vi "Retrieve trace.vi"(5 "max points":i32, 7 "Data.PG in":refnum<class "Data.PG.lvclass">, 8 "error in (no error)":errorcluster, 9 "path table:column":string, 10 "End":timestamp, 11 "Start":timestamp) -> (0 "error out":errorcluster, 2 "Trace":cluster{timestamp[], dbl[]}, 3 "Data.PG out":refnum<class "Data.PG.lvclass">)   [LabVIEW 2020, in "Data.PG.lvclass"]
uses:
  Data.PG.lvclass
  <vilib>/Utility/error.llb/Error Cluster From Error Code.vi
  <vilib>/ErrorRing/Error Ring.xnode
panel:
  out "resulting string":string
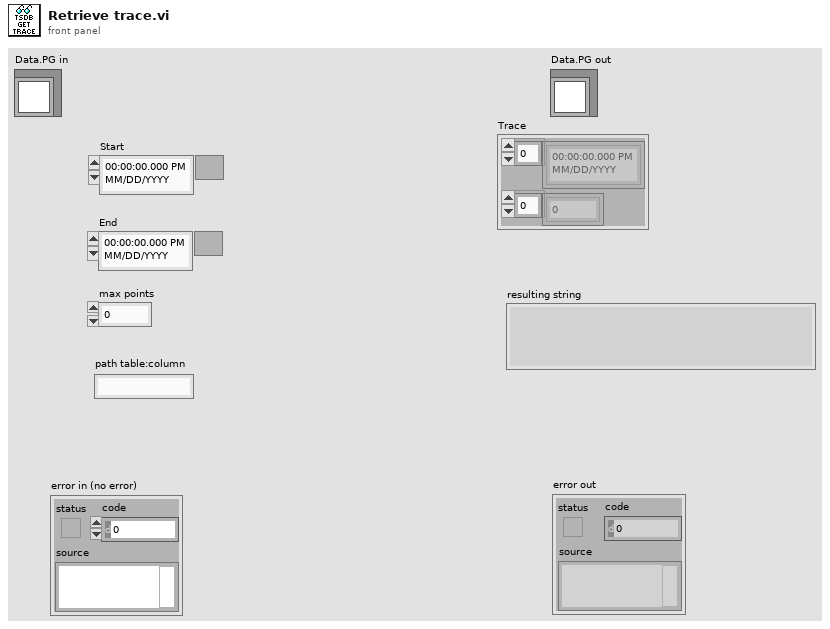
[diagram p1: front panel]
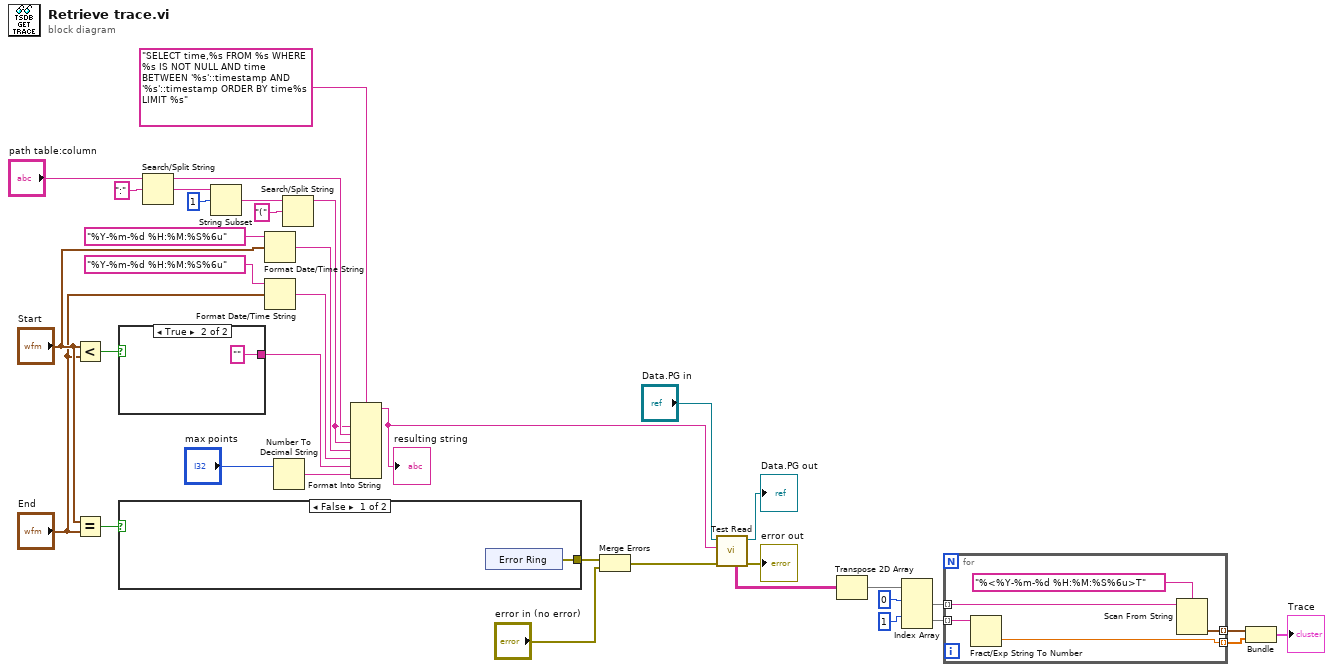
[diagram p0: block diagram]
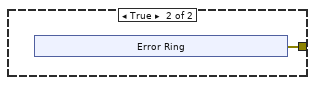
[diagram p2: hidden frame]
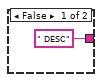
[diagram p3: hidden frame]
diagram:
  n1 = Less?(x="Start", y="End") -> (x < y?=w33:bool)
  n2 = Equal?(x="Start", y="End") -> (x = y?=w32:bool)
  n3 = case shown="True" w33 {
    tunnel: [" DESC" ""] -> w11
    frame False {
    }
    frame True {
    }
  }
  n4 = case shown="False" w32 {
    tunnel: [w39 w41] -> w31
    frame False {
      n5 = xnode "Error Ring"() -> ("error out"=w39:errorcluster)
    }
    frame True {
      n6 = xnode "Error Ring"() -> ("error out"=w41:errorcluster)
    }
  }
  n7 = Search/Split String(string="path table:column", search string/char (-)=":") -> (substring before match=w2:string, match + rest of string=w6:string)  [unwired: 1 in, 1 out]
  n8 = String Subset(string=w6, offset (0)=1) -> (substring=w4:string)  [unwired: 1 in]
  n9 = Format Date/Time String(time format string (%c)="%Y-%m-%d %H:%M:%S%6u", seconds (now)="Start") -> (date/time string=w9:string)  [unwired: 1 in]
  n10 = Format Date/Time String(time format string (%c)="%Y-%m-%d %H:%M:%S%6u", seconds (now)="End") -> (date/time string=w10:string)  [unwired: 1 in]
  n11 = Number To Decimal String(number="max points") -> (decimal integer string=w12:string)  [unwired: 1 in]
  n12 = Search/Split String(string=w4, search string/char (-)="(") -> (substring before match=w1:string)  [unwired: 1 in, 2 out]
  n13 = Format Into String(format string="SELECT time,%s FROM %s WHERE %s IS NOT NULL AND time BETWEEN '%s'::timestamp AND '%s'::timestamp ORDER BY time%s LIMIT %s", w1, w2, w1, w9, w10, w11, w12) -> (resulting string=w13:string)  [unwired: 2 in, 1 out]
  "resulting string" <- w13
  n14 = Merge Errors(w31, "error in (no error)") -> (w29:errorcluster)
  n15 = call-dynamic "Test Read.vi"("error in (no error)"=w29, "command"=w13, "Data.PG in"="Data.PG in") -> ("error out"=→"error out":errorcluster, "Data.PG out"=→"Data.PG out":refnum<class "Data.PG.lvclass">, "Result"=w28:string[][])  [unwired: 3 in, 3 out]
  n16 = Transpose 2D Array(2D array=w28) -> (transposed array=w27:string[][])
  n17 = Index Array(array=w27, index (row) #1=0 ("index (row)"), index (row) #2=1 ("index (row)")) -> (element #1=w24:string[], element #2=w23:string[])  [unwired: 2 in]
  n18 = for {
    tunnel: w24 -> [w50] mode=indexing
    tunnel: w23 -> [w49] mode=indexing
    tunnel: [w48] -> w21 mode=indexing
    tunnel: [w47] -> w22 mode=indexing
    n19 = Fract/Exp String To Number(string=w49) -> (number=w48:dbl)  [unwired: 3 in, 1 out]
    n20 = Scan From String(format string="%<%Y-%m-%d %H:%M:%S%6u>T", input string=w50) -> (output 1=w47:timestamp)  [unwired: 3 in, 3 out]
  }
  n21 = Bundle(w22, w21) -> (→"Trace":cluster{timestamp[], dbl[]})  [unwired: 1 in]
